vi "testApplication.vi"(11 "Settings":T1={"IP"="140.252.32.156", "port_low"=9999, "port_up"=9999, "connection_timeout "=1500, "reading_timeout"=1500, "writing_timeout"=1500}) -> ()   [LabVIEW 2016]
uses:
  ts_labview_tcp/tcpTypedefs/TCPSettings.ctl
  ts_labview_tcp/TCPSettings/TCPSettings.lvclass
  ts_labview_tcp/TCPClient/TCPClient.lvclass
  home/harini/tcs/ss_SpectrographInstrument/ts_labview_tcp/TCPCommunicator/TCPCommunicator.lvclass
  SpectrographClientCommunicator/SpectrographClientCommunicator.lvclass
  ts_labview_tcp/TCPCommunicator/TCPCommunicator.lvclass/TCPCommunicator.ctl
  ts_labview_tcp/TCPComEvents/TCPComEvents.lvclass
  ts_labview_tcp/TCPCommunicator/TCPCommunicator.lvclass
panel:
  out "Output":string
  out "Filter Wheel Position":u8
  in  "getFilterWheelPosition":bool
  in  "stop":bool
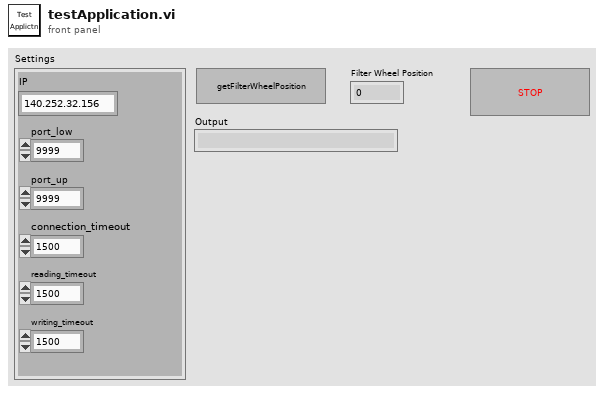
[diagram p1: front panel]
types:
  T1 = typedef "TCPSettings.ctl" = cluster{"IP":string, "port_low":u16, "port_up":u16, "connection_timeout ":i32, "reading_timeout":i32, "writing_timeout":i32}
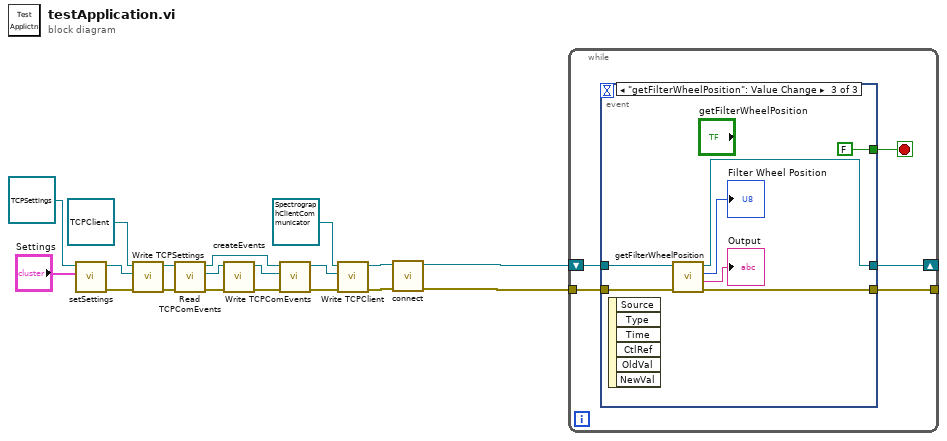
[diagram p0: block diagram]
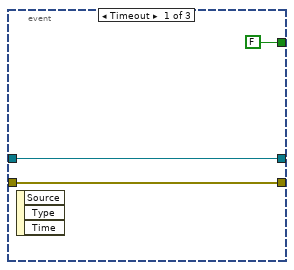
[diagram p2: hidden frame]
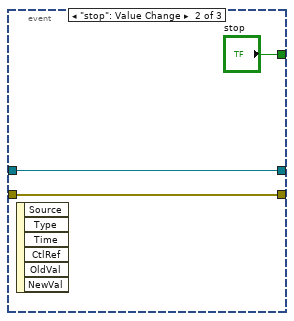
[diagram p3: hidden frame]
diagram:
  n1 = call "setSettings.vi"("Settings"="Settings", "TCPSettings in"=refnum<class "TCPSettings.lvclass"> refnum ("TCPSettings.lvclass")) -> ("error out"=w15:errorcluster, "TCPSettings out"=w16:refnum<class "TCPSettings.lvclass">)  [unwired: 8 in]
  n2 = call-dynamic "Write TCPSettings.vi"("error in (no error)"=w15, "TCPSettings.lvclass"=w16, "TCPCommunicator in"=refnum<class "TCPClient.lvclass"> refnum ("TCPClient.lvclass")) -> ("error out"=w10:errorcluster, "TCPCommunicator out"=w14:refnum<class "TCPClient.lvclass">)  [unwired: 7 in]
  n3 = call "Read TCPComEvents.vi"("error in (no error)"=w10, "TCPCommunicator in"=w14) -> ("error out"=w9:errorcluster, "TCPComEvents.lvclass"=w13:refnum<class "TCPComEvents.lvclass">, "TCPCommunicator out"=w11:refnum<class "TCPClient.lvclass">)  [unwired: 7 in]
  n4 = call "createEvents.vi"("error in (no error)"=w9, "TCPComEvents in"=w13) -> ("error out"=w8:errorcluster, "TCPComEvents out"=w12:refnum<class "TCPComEvents.lvclass">)  [unwired: 8 in]
  n5 = call "Write TCPComEvents.vi"("error in (no error)"=w8, "TCPComEvents.lvclass"=w12, "TCPCommunicator in"=w11) -> ("error out"=w5:errorcluster, "TCPCommunicator out"=w6:refnum<class "TCPClient.lvclass">)  [unwired: 7 in]
  n6 = call-dynamic "Write TCPClient.vi"("error in (no error)"=w5, "TCPClient"=w6, "SpectrographClientCommunicator in"=refnum<class "SpectrographClientCommunicator.lvclass"> refnum ("SpectrographClientCommunicator.lvclass")) -> ("error out"=w3:errorcluster, "SpectrographClientCommunicator out"=w4:refnum<class "SpectrographClientCommunicator.lvclass">)  [unwired: 7 in]
  n7 = call "connect.vi"("error in (no error)"=w3, "SpectrographClientCommunicator in"=w4) -> ("error out"=w1:errorcluster, "SpectrographClientCommunicator out"=w2:refnum<class "SpectrographClientCommunicator.lvclass">)  [unwired: 8 in]
  n8 = while {
    tunnel: w1 -> [w24]
    shift-right: [w22] -> _
    shift-left: w2 -> [w23]
    tunnel: [w20] -> _
    stop <- w21 stop-if-true
    n9 = event shown="[2] \"getFilterWheelPosition\": Value Change" {
      selector: _ -> [_ _ _]
      dyn-events: _ -> [_ _ _]
      timeout: _ -> [_ _ _]
      tunnel: [w26 w28 w35] -> w20
      tunnel: w24 -> [w26 w28 w36]
      tunnel: w23 -> [w27 w30 w37]
      tunnel: [w27 w30 w34] -> w22
      tunnel: [FALSE ("stop") "stop" FALSE ("stop")] -> w21
      event Timeout {
        n10 = event-data() -> ()  [unwired: 1 in, 3 out]
      }
      event "stop": Value Change {
        n11 = event-data() -> ()  [unwired: 1 in, 6 out]
      }
      event "getFilterWheelPosition": Value Change {
        n12 = event-data() -> ()  [unwired: 1 in, 6 out]
        n13 = call "getFilterWheelPosition.vi"("error in (no error)"=w36, "SpectrographClientCommunicator in"=w37) -> ("error out"=w35:errorcluster, "Output"=→"Output":string, "Filter Wheel Position"=→"Filter Wheel Position":u8, "SpectrographClientCommunicator out"=w34:refnum<class "SpectrographClientCommunicator.lvclass">)  [unwired: 6 in]
      }
    }
  }
